vi "ezAFM Practice 1.9.vi"() -> ()   [LabVIEW 2015]
uses:
  LabVIEW for ezAFM/LV-PGC 2019-05a/Universal vi's/Controls/RoboProbe/RoboProbe ID.ctl
  LabVIEW for ezAFM/LV-PGC 2019-05a/Universal vi's/Controls/RoboProbe/RoboProbe PadResults.ctl
  LabVIEW for ezAFM/LV-PGC 2019-05a/Universal vi's/Controls/RoboProbe/RoboProbe DeviceTypes.ctl
  <vilib>/userdefined/High Color/IMAQdx.ctl
  D:/LabVIEW for ezAFM/LV-PGC 2019-05a/Special Equipment/ezAFM/NMI Integration Code/ezCommander.dll
  LabVIEW for ezAFM/LV-PGC 2019-05a/Special Equipment/ezAFM/NMI Integration Code/ezCommander.dll
  LabVIEW for ezAFM/LV-PGC 2019-05a/Universal vi's/Global Variables/Globals-EasyAFM.vi
  Helper VI's/Globals.vi
  <vilib>/vision/driver/NI_Vision_Acquisition_Software.lvlib
panel:
  in  "Update Device List":bool
  out "List of Connections":string[](array[string])
  out "Selected \nConnections":T1[](array[typedef]) {"Results"."Rpad" format="%_2e"; "Results"."S" format="%_2g"; "Results"."Vt" format="%.1f"; "Results"."DV" format="%.2g"; "Results"."Ron" format="%.2e"; "Results"."Roff" format="%.2g"; "Results"."Vg-off" format="%.2g"; "Results"."Vg-on" format="%.2g"; "Results"."DG%" format="%.1f"; "Results"."Gon" format="%.2e"; "Results"."Goff" format="%.2e"; "Results"."Rgate" format="%.2e"; "Results"."I offset" format="%.2e"; "G(Vg)" format="%#_2e"; "ID"."Die" items=["AD", "AE", "AF", "AG", "AH", "AI", "AJ", "BC", "BD", "BE", "BF", "BG", "BH", "BI", "BJ", "BK", "CB", "CC", "CD", "CE", "CF", "CG", "CH", "CI", "CJ", "CK", "CL", "DA", "DB", "DC", "DD", "DE", "DF", "DG", "DH", "DI", "DJ", "DK", "DL", "DM", "EA", "EB", "EC", "ED", "EE", "EF", "EG", "EH", "EI", "EJ", "EK", "EL", "EM", "FA", "FB", "FC", "FD", "FE", "FF", "FG", "FH", "FI", "FJ", "FK", "FL", "FM", "GA", "GB", "GC", "GD", "GE", "GF", "GG", "GH", "GI", "GJ", "GK", "GL", "GM", "HA", "HB", "HC", "HD", "HE", "HF", "HG", "HH", "HI", "HJ", "HK", "HL", "HM", "IA", "IB", "IC", "ID", "IE", "IF", "IG", "IH", "II", "IJ", "IK", "IL", "IM", "JB", "JC", "JD", "JE", "JF", "JG", "JH", "JI", "JJ", "JK", "JL", "KC", "KD", "KE", "KF", "KG", "KH", "KI", "KJ", "KK", "LD", "LE", "LF", "LG", "LH", "LI", "LJ"]; "ID"."Leads" items=["ab", "bc", "cd", "de", "ef", "fg", "gh", "ac", "ce", "eg", "bd", "df", "fh"]; "ID"."Device#" items=["00", "01", "02", "03", "10", "11", "12", "13", "20", "21", "22", "23", "30", "31", "32", "33"]; "Date" format="%<%H:%M\n%d/%m/%y>T"}
  out "Scan Spot Coordinates":dbl[](array[numeric])
  out "Name":string
  out "Sequence Index":dbl
  out "Direction":dbl
  out "Crosshair Found?":bool
  in  "Search":bool
  out "Total Steps":dbl
  out "Current Steps":dbl
  in  "Camera":enum32{"ezAFM Camera"}(tab)
  out "ezAFM Camera":T4(plugin-control)
  in  "Connection to Scan":string
  in  "Initialize Automatic \nRepositioning":bool
  out "Imaging Status":string
  out "Automated Imaging":bool
  in  "Main Menu":T5(tab)
  in  "Navigation Buttons":T6
  in  "Motor Speed":u16(ring)=30000 items=["SLOW"=3300, "MEDIUM"=30000, "FAST"=65000]
  in  "Target Crosshair":string(combo)="00 | 01"
  in  "Current Crosshair":string(combo)="00 | 01"
  in  "MOVE2CROSSHAIR":bool
  in  "THETA":bool
  in  "Angle":dbl
  in  "Step Size":dbl
  in  "Scan Spot":string(combo)
  in  "MOVE2SCANSPOT":bool
  in  "RETRACT":bool
  in  "APPROACH":bool
  in  "SEARCH":bool
  in  "SCAN":bool
  in  "REMOVE":bool
  out "Sequence":string[](array[string])
  in  "Initialize Automated Imaging":bool
  in  "SELECT":bool
  in  "DeviceList":i32(listbox) caption="Devices Selected for AFM Imaging"
  in  "ezAFM Default File Path":path=path "D:/ezAFM/Scanned Images"
  in  "Saved Images File Path":path=path "D:/ezAFM/Scanned Images"
  in  "Wafer Type":string(combo)
  in  "Die":string(combo)
  in  "Image Resolution":u16(ring)=256 items=["128"=128, "256"=256, "512"=512, "1024"=1024]
  in  "Indicators":enum32{"Indicators"}(tab)
  out "XYZ Motor Position":dbl[](array[numeric]) format="%#_4f"
  out "ezAFM Status":dbl
  out "Approaching":bool
  out "ezAFM Connected":bool
  out "Retracting":bool
  out "Scanning":bool
  out "Tip Approached?":bool
  in  "RESET":bool
  out "XY Position":dbl[](array[numeric])
  in  "QUIT":bool
  out "Searching":bool
  # "ON"
  # "OFF"
  # "Use Arrow Keys to manually\nmove the XY Motor"
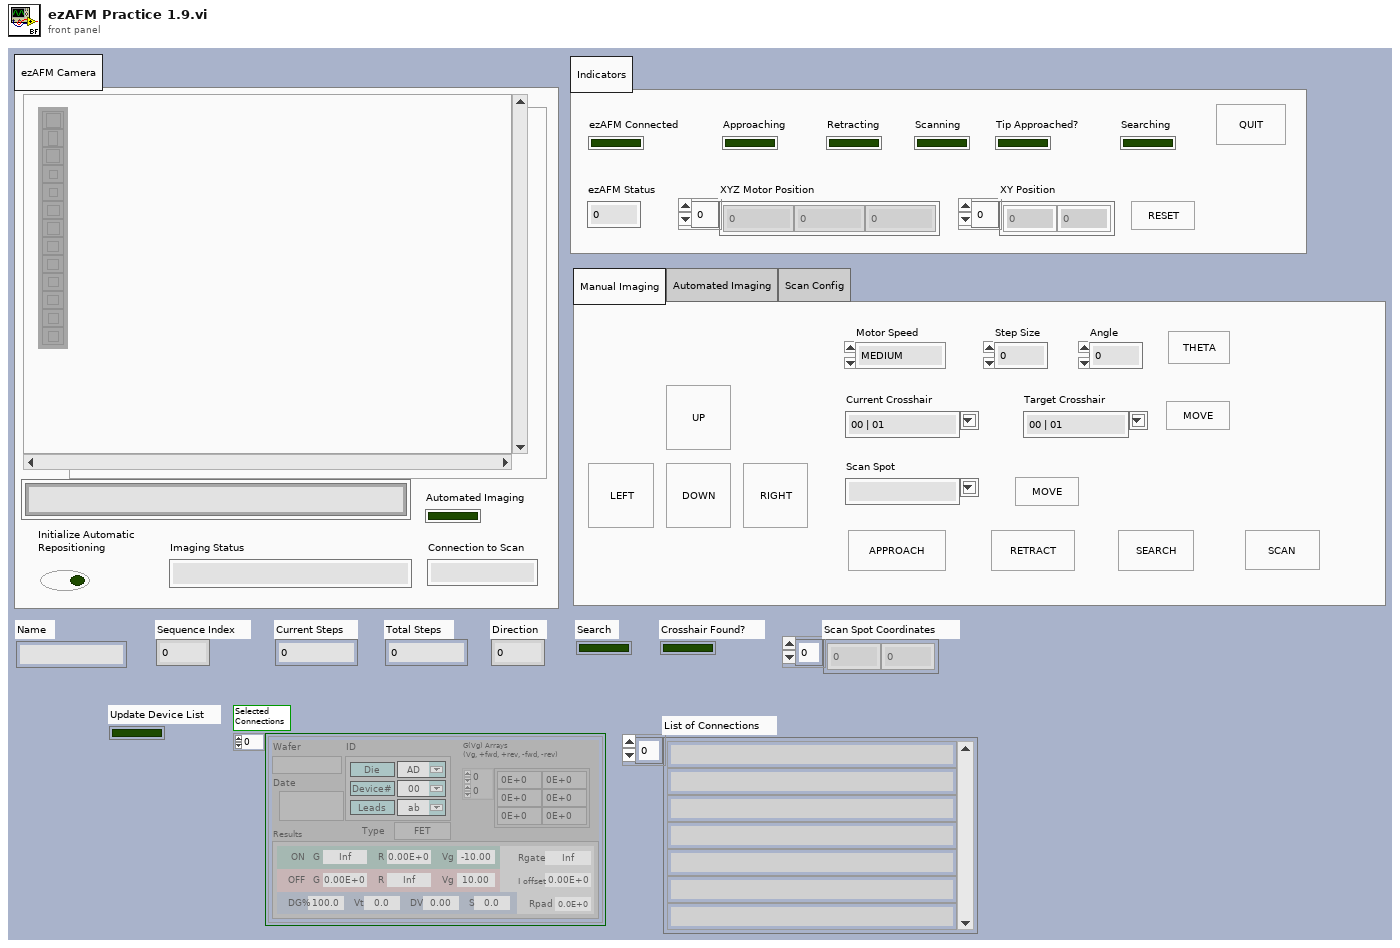
[diagram p1: front panel]
types:
  T1 = typedef "RoboProbe ID.ctl" = cluster{"Wafer":string, "Date":timestamp, "ID":cluster{"Device#":u16, "Leads":u16, "Die":u16}, "G(Vg)":sgl[][], "Results":T2, "Type":T3}
  T2 = typedef "RoboProbe PadResults.ctl" = cluster{"I offset":sgl, "Rgate":sgl, "Gon":sgl, "Goff":sgl, "DG%":sgl, "Ron":sgl, "Vg-on":sgl, "Roff":sgl, "Vg-off":sgl, "DV":sgl, "Vt":sgl, "S":sgl, "Rpad":sgl}
  T3 = typedef "RoboProbe DeviceTypes.ctl" = enum16{"FET", "Metal", "Mixed", "GateLeak", "ShortCirc", "Open", "Untested"}
  T4 = typedef "IMAQ Image.ctl" = refnum<image>
  T5 = enum32{"Manual Imaging", "Automated Imaging", "Scan Config"}
  T6 = cluster{"UP":bool, "DOWN":bool, "LEFT":bool, "RIGHT":bool}
  T7 = typedef "IMAQdx.ctl" = refnum<k21>
  T8 = typedef "Image Type" = u32
  T9 = typedef "eventvkey.ctl" = enum16{"ASCII", "Enter", "Return", "Shift", "Ctrl", "Alt", "Cmd", "Opt", "Caps", "NumLock", "Clear", "Break", "Up", "Down", "Left", "Right", "Insert", "Delete", "Home", "End", "PageUp", "PageDown", "Escape", "Help", "Pause", "ScrollLock", "F1", "F2", "F3", "F4", "F5", "F6", "F7", "F8", "F9", "F10", "F11", "F12", "F13", "F14", "F15", "F16", "F17", "F18", "F19", "F20", "F21", "F22", "F23", "F24", "Play", "VolumeUp", "VolumeDown", "Mute", "Two Byte Char"}
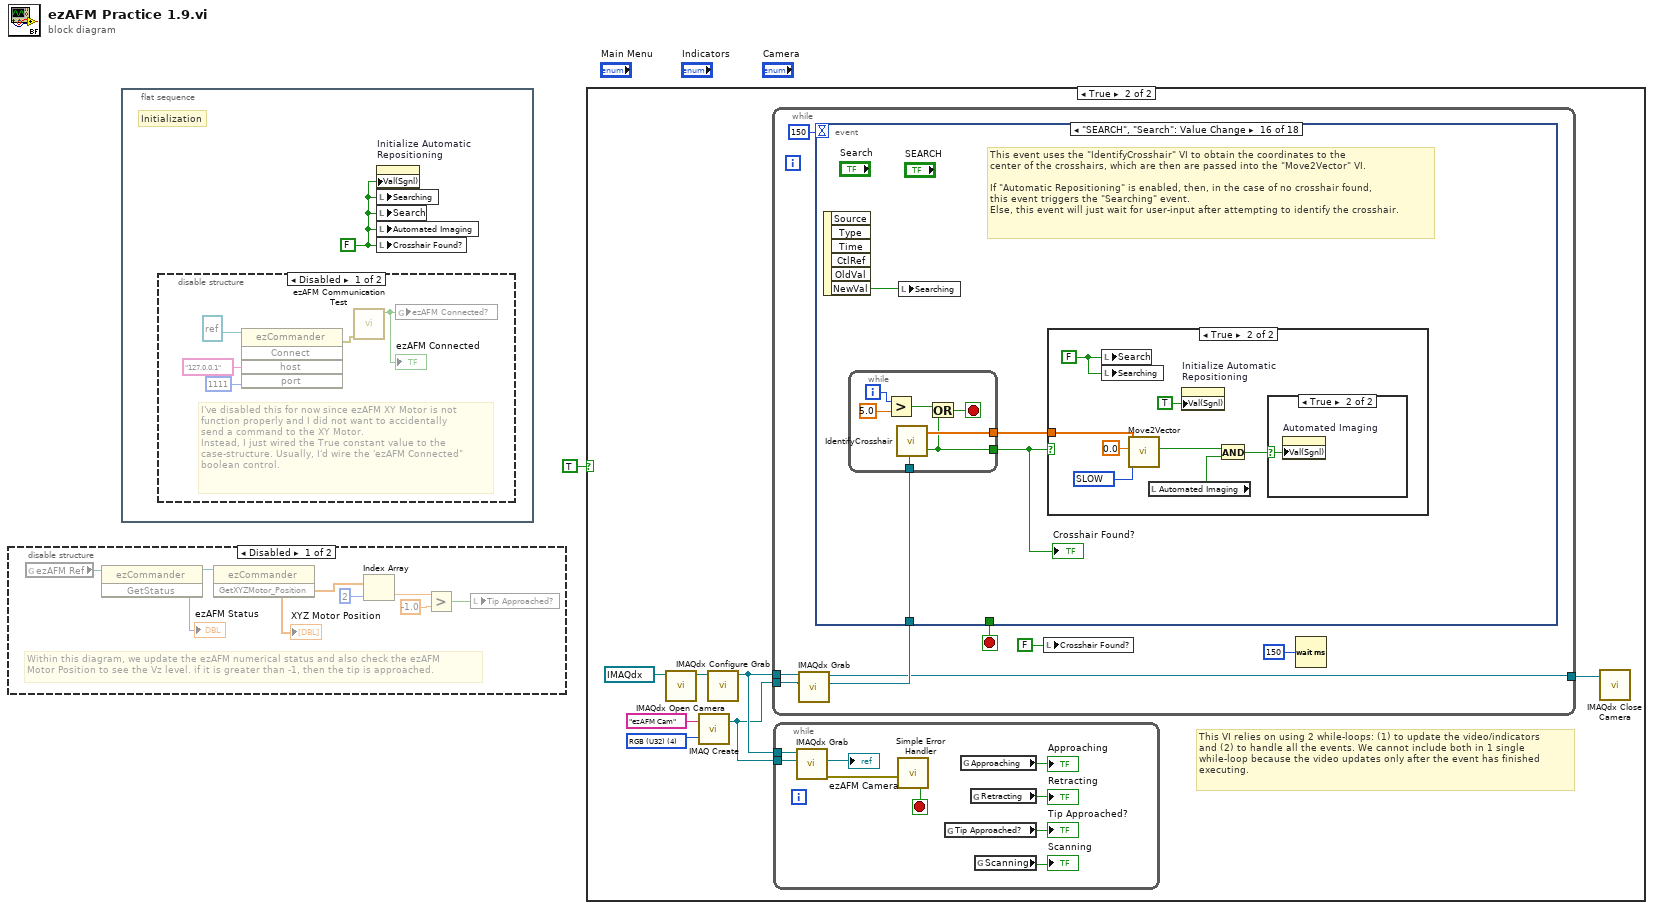
[diagram p0: block diagram]
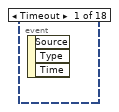
[diagram p5: hidden frame]
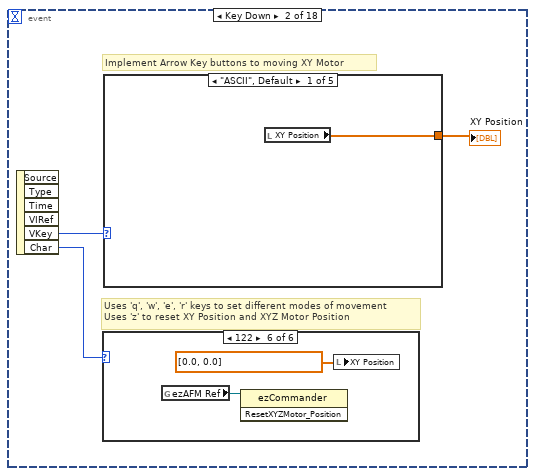
[diagram p6: hidden frame]
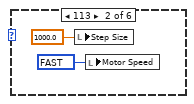
[diagram p8: hidden frame]
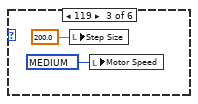
[diagram p9: hidden frame]
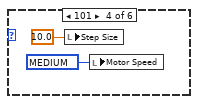
[diagram p10: hidden frame]
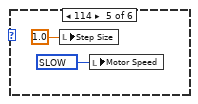
[diagram p11: hidden frame]
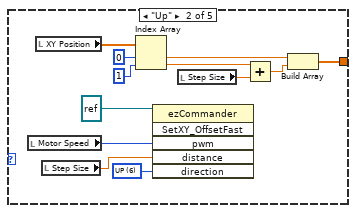
[diagram p12: hidden frame]
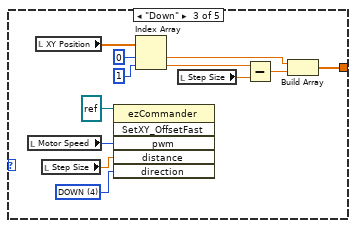
[diagram p13: hidden frame]
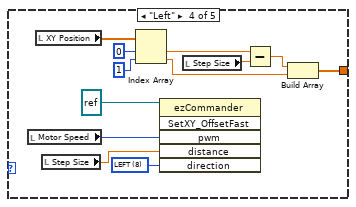
[diagram p14: hidden frame]
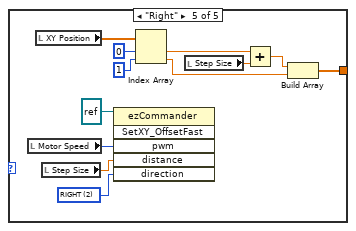
[diagram p15: hidden frame]
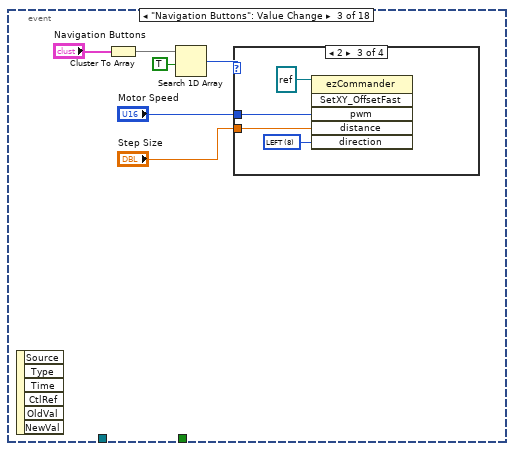
[diagram p16: hidden frame]
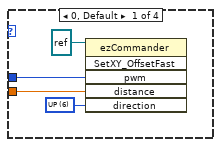
[diagram p17: hidden frame]
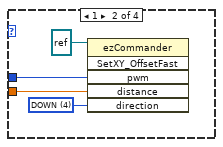
[diagram p18: hidden frame]
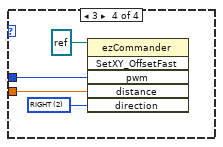
[diagram p19: hidden frame]
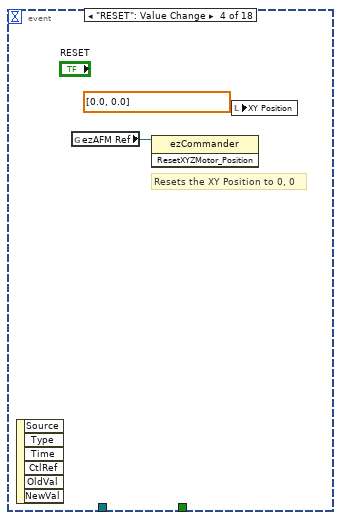
[diagram p20: hidden frame]
diagram:
  n1 = disable-structure shown="Disabled" {
    frame Disabled {
      # "Within this diagram, we update the ezAFM numerical status and also check the ezAFM\nMotor Position to see the Vz level. if it is greater than -1, then the tip is approached."
      n2 = global read "Globals-EasyAFM.vi" "ezAFM Ref"() -> (w7:refnum<k24>)
      n3 = invoke class="ezCommander" method="GetStatus"(reference=w7) -> (reference out=w5:refnum<k24>, "GetStatus"=→"ezAFM Status":i32)  [unwired: 2 in, 1 out]
      n4 = invoke class="ezCommander" method="GetXYZMotor_Position"(reference=w5) -> ("GetXYZMotor_Position"=w9:dbl[])  [unwired: 2 in, 2 out]
      "XYZ Motor Position" <- w9
      n5 = Index Array(array=w9, index=2) -> (element=w4:dbl)
      n6 = Greater?(x=w4, y=-1.0) -> (0:w8:bool)
      n7 = local write "Tip Approached?"(w8) -> ()
    }
    frame Enabled {
    }
  }
  n8 = flat-sequence {
    frame #0 {
      w10 = FALSE ("Automated Imaging")
      # "Initialization"
      n9 = disable-structure shown="Disabled" {
        frame Disabled {
          # "I've disabled this for now since ezAFM XY Motor is not \nfunction properly and I did not want to accidentally\nsend a command to the XY Motor. \nInstead, I just wired the True constant value to the \ncase-structure. Usually, I'd wire the 'ezAFM Connected\"\nboolean control."
          n10 = invoke class="ezCommander" method="Connect"(reference=refnum<k24> refnum ("ezAFM Ref"), "host"="127.0.0.1", "port"=1111) -> (error out=w14:errorcluster)  [unwired: 2 in, 4 out]
          n11 = call "ezAFM Communication Test.vi"("error in"=w14) -> ("ezAFM COM status"=w11:bool)  [unwired: 3 in, 3 out]
          "ezAFM Connected" <- w11
          n12 = global write "Globals.vi" "ezAFM Connected?"(w11) -> ()
        }
        frame Enabled {
        }
      }
      n13 = property on="Initialize Automatic \nRepositioning" class="Bool (strict)"("Val(Sgnl)"=w10) -> ()  [unwired: 2 in, 2 out]
      n14 = local write "Searching"(w10) -> ()
      n15 = local write "Search"(w10) -> ()
      n16 = local write "Automated Imaging"(w10) -> ()
      n17 = local write "Crosshair Found?"(w10) -> ()
    }
  }
  n18 = case shown="True" TRUE {
    frame False {
    }
    frame True {
      w19 = T8 4 items=["Grayscale (U8)", "Grayscale (I16)", "Grayscale (SGL)", "Complex (CSG)", "RGB (U32)", "HSL (U32)", "RGB (U64)", "Grayscale (U16)"] ("Image Type")
      # "This VI relies on using 2 while-loops: (1) to update the video/indicators \nand (2) to handle all the events. We cannot include both in 1 single \nwhile-loop because the video updates only after the event has finished \nexecuting."
      n19 = call <vilib>:"IMAQdx Open Camera.vi"("Session In"=T7 "cam5") -> ("Session Out"=w20:T7)  [unwired: 9 in, 1 out]
      n20 = call "IMAQ Create"("Image Name"="ezAFM Cam", "Image Type"=w19) -> ("New Image"=w17:T4)  [unwired: 3 in, 1 out]
      n21 = call <vilib>:"IMAQdx Configure Grab.vi"("Session In"=w20) -> ("Session Out"=w18:T7)  [unwired: 9 in, 1 out]
      n22 = while {
        tunnel: w18 -> [w37]
        tunnel: w17 -> [w36]
        tunnel: [w34] -> w16
        stop <- w33 stop-if-true
        n23 = call <vilib>:"IMAQdx Grab.vi"("Image In"=w36, "Session In"=w37) -> ("Image Out"=w35:T4, "Session Out"=w34:T7)  [unwired: 2 in, 6 out]
        n24 = event shown="[15] \"SEARCH\", \"Search\": Value Change" {
          selector: _ -> [_ _ _ _ _ _ _ _ _ _ _ _ _ _ _ _ _ _]
          dyn-events: _ -> [_ _ _ _ _ _ _ _ _ _ _ _ _ _ _ _ _ _]
          timeout: 150 -> [_ _ _ _ _ _ _ _ _ _ _ _ _ _ _ _ _ _]
          tunnel: [_ _ _ _ _ _ _ _ _ _ _ _ _ _ _ _ _ "QUIT"] -> w33
          tunnel: w35 -> [_ _ _ _ _ _ _ _ _ _ _ _ _ _ _ w307 _ _]
          event Timeout {
            n25 = event-data() -> ()  [unwired: 1 in, 3 out]
          }
          event Key Down {
            # "Uses 'q', 'w', 'e', 'r' keys to set different modes of movement\nUses 'z' to reset XY Position and XYZ Motor Position"
            # "Implement Arrow Key buttons to moving XY Motor"
            n26 = event-data() -> ("VKey"=w40:T9, "Char"=w41:i16)  [unwired: 1 in, 4 out]
            n27 = case shown="122" w41 {
              frame 0, Default {
              }
              frame 113 {
                w43 = u16 65000 items=["SLOW"=3300, "MEDIUM"=30000, "FAST"=65000] ("Motor Speed")
                n28 = local write "Step Size"(1000.0 ("Step Size")) -> ()
                n29 = local write "Motor Speed"(w43) -> ()
              }
              frame 119 {
                w45 = u16 30000 items=["SLOW"=3300, "MEDIUM"=30000, "FAST"=65000] ("Motor Speed")
                n30 = local write "Step Size"(200.0 ("Step Size")) -> ()
                n31 = local write "Motor Speed"(w45) -> ()
              }
              frame 101 {
                w47 = u16 30000 items=["SLOW"=3300, "MEDIUM"=30000, "FAST"=65000] ("Motor Speed")
                n32 = local write "Step Size"(10.0 ("Step Size")) -> ()
                n33 = local write "Motor Speed"(w47) -> ()
              }
              frame 114 {
                w49 = u16 3300 items=["SLOW"=3300, "MEDIUM"=30000, "FAST"=65000] ("Motor Speed")
                n34 = local write "Step Size"(1.0 ("Step Size")) -> ()
                n35 = local write "Motor Speed"(w49) -> ()
              }
              frame 122 {
                n36 = global read "Globals-EasyAFM.vi" "ezAFM Ref"() -> (w51:refnum<k24>)
                n37 = invoke class="ezCommander" method="ResetXYZMotor_Position"(reference=w51) -> ()  [unwired: 2 in, 3 out]
                n38 = local write "XY Position"(dbl[] [0.0, 0.0] ("XY Position")) -> ()
              }
            }
            n39 = case shown="\"ASCII\", Default" w40 {
              tunnel: [w53 w55 w66 w78 w90] -> w42
              frame "ASCII", Default {
                n40 = local read "XY Position"() -> (w53:dbl[])
              }
              frame "Up" {
                w64 = u16 6 items=["UP"=6, "DOWN"=4, "LEFT"=8, "RIGHT"=2]
                n41 = local read "Motor Speed"() -> (w63:u16)
                n42 = local read "XY Position"() -> (w61:dbl[])
                n43 = local read "Step Size"() -> (w62:dbl)
                n44 = Index Array(array=w61, index #1=0 ("index"), index #2=1 ("index")) -> (element #1=w57:dbl, element #2=w54:dbl)
                n45 = invoke class="ezCommander" method="SetXY_OffsetFast"(reference=refnum<k24> refnum ("ezAFM Ref"), "pwm"=w63, "distance"=w62, "direction"=w64) -> ()  [unwired: 2 in, 6 out]
                n46 = local read "Step Size"() -> (w58:dbl)
                n47 = Add(x=w54, y=w58) -> (x+y=w56:dbl)
                n48 = Build Array(w57, w56) -> (w55:dbl[])
              }
              frame "Down" {
                w74 = u16 4 items=["UP"=6, "DOWN"=4, "LEFT"=8, "RIGHT"=2]
                n49 = local read "Motor Speed"() -> (w76:u16)
                n50 = local read "XY Position"() -> (w68:dbl[])
                n51 = local read "Step Size"() -> (w75:dbl)
                n52 = invoke class="ezCommander" method="SetXY_OffsetFast"(reference=refnum<k24> refnum ("ezAFM Ref"), "pwm"=w76, "distance"=w75, "direction"=w74) -> ()  [unwired: 2 in, 6 out]
                n53 = Index Array(array=w68, index #1=0 ("index"), index #2=1 ("index")) -> (element #1=w70:dbl, element #2=w71:dbl)
                n54 = local read "Step Size"() -> (w67:dbl)
                n55 = Subtract(x=w71, y=w67) -> (x-y=w69:dbl)
                n56 = Build Array(w70, w69) -> (w66:dbl[])
              }
              frame "Left" {
                w88 = u16 8 items=["UP"=6, "DOWN"=4, "LEFT"=8, "RIGHT"=2]
                n57 = local read "Motor Speed"() -> (w86:u16)
                n58 = local read "XY Position"() -> (w82:dbl[])
                n59 = local read "Step Size"() -> (w87:dbl)
                n60 = Index Array(array=w82, index #1=0 ("index"), index #2=1 ("index")) -> (element #1=w81:dbl, element #2=w79:dbl)
                n61 = invoke class="ezCommander" method="SetXY_OffsetFast"(reference=refnum<k24> refnum ("ezAFM Ref"), "pwm"=w86, "distance"=w87, "direction"=w88) -> ()  [unwired: 2 in, 6 out]
                n62 = local read "Step Size"() -> (w83:dbl)
                n63 = Subtract(x=w81, y=w83) -> (x-y=w80:dbl)
                n64 = Build Array(w80, w79) -> (w78:dbl[])
              }
              frame "Right" {
                w100 = u16 2 items=["UP"=6, "DOWN"=4, "LEFT"=8, "RIGHT"=2]
                n65 = local read "Motor Speed"() -> (w99:u16)
                n66 = local read "XY Position"() -> (w95:dbl[])
                n67 = local read "Step Size"() -> (w98:dbl)
                n68 = invoke class="ezCommander" method="SetXY_OffsetFast"(reference=refnum<k24> refnum ("ezAFM Ref"), "pwm"=w99, "distance"=w98, "direction"=w100) -> ()  [unwired: 2 in, 6 out]
                n69 = Index Array(array=w95, index #1=0 ("index"), index #2=1 ("index")) -> (element #1=w93:dbl, element #2=w91:dbl)
                n70 = local read "Step Size"() -> (w94:dbl)
                n71 = Add(x=w93, y=w94) -> (x+y=w92:dbl)
                n72 = Build Array(w92, w91) -> (w90:dbl[])
              }
            }
            "XY Position" <- w42
          }
          event "Navigation Buttons": Value Change {
            n73 = event-data() -> ()  [unwired: 1 in, 6 out]
            n74 = Cluster To Array(cluster="Navigation Buttons") -> (array=w106:bool[])
            n75 = Search 1D Array(1D array=w106, element=TRUE) -> (index of element=w104:i32)  [unwired: 1 in]
            n76 = case shown="2" w104 {
              tunnel: "Step Size" -> [w108 w113 w117 w121]
              tunnel: "Motor Speed" -> [w109 w112 w116 w120]
              frame 0, Default {
                w110 = u16 6 items=["UP"=6, "DOWN"=4, "LEFT"=8, "RIGHT"=2]
                n77 = invoke class="ezCommander" method="SetXY_OffsetFast"(reference=refnum<k24> refnum ("ezAFM Ref"), "pwm"=w109, "distance"=w108, "direction"=w110) -> ()  [unwired: 2 in, 6 out]
              }
              frame 1 {
                w114 = u16 4 items=["UP"=6, "DOWN"=4, "LEFT"=8, "RIGHT"=2]
                n78 = invoke class="ezCommander" method="SetXY_OffsetFast"(reference=refnum<k24> refnum ("ezAFM Ref"), "pwm"=w112, "distance"=w113, "direction"=w114) -> ()  [unwired: 2 in, 6 out]
              }
              frame 2 {
                w118 = u16 8 items=["UP"=6, "DOWN"=4, "LEFT"=8, "RIGHT"=2]
                n79 = invoke class="ezCommander" method="SetXY_OffsetFast"(reference=refnum<k24> refnum ("ezAFM Ref"), "pwm"=w116, "distance"=w117, "direction"=w118) -> ()  [unwired: 2 in, 6 out]
              }
              frame 3 {
                w122 = u16 2 items=["UP"=6, "DOWN"=4, "LEFT"=8, "RIGHT"=2]
                n80 = invoke class="ezCommander" method="SetXY_OffsetFast"(reference=refnum<k24> refnum ("ezAFM Ref"), "pwm"=w120, "distance"=w121, "direction"=w122) -> ()  [unwired: 2 in, 6 out]
              }
            }
          }
          event "RESET": Value Change {
            # "Resets the XY Position to 0, 0"
            n81 = event-data() -> ()  [unwired: 1 in, 6 out]
            n82 = global read "Globals-EasyAFM.vi" "ezAFM Ref"() -> (w124:refnum<k24>)
            n83 = invoke class="ezCommander" method="ResetXYZMotor_Position"(reference=w124) -> ()  [unwired: 2 in, 3 out]
            n84 = local write "XY Position"(dbl[] [0.0, 0.0] ("XY Position")) -> ()
          }
          event "THETA": Value Change {
            # "NOTE: 9/17/2019: This feature does not work reliably because XY Position is a simple record of horizontal\nand vertical movements without accounting for Motor Speed. Different Motor Speeds lead to different\nerror and physical distance values.\nI've noticed that using any generic angle measurement tool such as Windows Snip and entering the estimated angle\ninto the control value works sufficiently."
            # "Takes the absolute value of the XY Position and computes the magnitude of the angle.\nThen based on the sign of the X and Y position, we change the sign of the angle\nIf both signs are the same, then the angle should be negative (clockwise rotated by theta)\nElse if both signs are different, then the angle should be positive (counter-clockwise rotated)"
            n85 = event-data() -> ()  [unwired: 1 in, 6 out]
            n86 = local read "XY Position"() -> (w139:dbl[])
            n87 = Absolute Value(x=w139) -> (abs(x)=w140:dbl[])
            n88 = Index Array(array=w139) -> (element #1=w133:dbl, element #2=w132:dbl)  [unwired: 2 in]
            n89 = Index Array(array=w140, index #1=1 ("index"), index #2=0 ("index")) -> (element #1=w136:dbl, element #2=w135:dbl)
            n90 = Re/Im To Complex(1:w135, 2:w136) -> (0:w134:cdb)
            n91 = Sign(1:w133) -> (0:w131:dbl)
            n92 = Sign(1:w132) -> (0:w130:dbl)
            n93 = Complex To Polar(r * e^(i*theta)=w134) -> (theta=w128:dbl)  [unwired: 1 out]
            n94 = Equal?(x=w131, y=w130) -> (x = y?=w129:bool)
            n95 = case shown="True" w129 {
              tunnel: w128 -> [w141 w143]
              tunnel: [w141 w142] -> w127
              frame False {
              }
              frame True {
                n96 = Negate(x=w143) -> (-x=w142:dbl)
              }
            }
            n97 = expression code="(x/pi)*180.0" "radians to degrees"(w127) -> (w126:dbl)
            n98 = local write "Angle"(w126) -> ()
            n99 = global write "Globals.vi" "THETA"(w126) -> ()
          }
          event "APPROACH", "RETRACT": Value Change {
            n100 = event-data() -> ()  [unwired: 1 in, 6 out]
            n101 = case shown="True" "APPROACH" {
              selector: "APPROACH" -> [_ w149]
              frame False {
              }
              frame True {
                n102 = call "AutoLand&Approach.vi"("Autoland?"=w149, "Step-Approach?"=FALSE) -> ()  [unwired: 1 out]
              }
            }
            n103 = case shown="True" "RETRACT" {
              selector: "RETRACT" -> [_ w146]
              frame False {
              }
              frame True {
                n104 = call "Retract.vi"("Number of Cycles"=10, "Retracting?"=w146) -> ()  [unwired: 1 out]
              }
            }
          }
          event "SELECT", "REMOVE": Value Change {
            # "This event handles selecting/removing connections to scan.\nI copied/pasted this from Trevor's \"ezAFM Automated Imaging 3.3\"\n\n10/6/2019: There are some file errors (\"Device Config\") with the \"SimpleMap\" VI"
            n105 = event-data() -> ()  [unwired: 1 in, 6 out]
            n106 = case shown="True" "SELECT" {
              frame False {
              }
              frame True {
                n107 = call "SimpleMap.vi"() -> ("Selected Connections"=→"Selected \nConnections":T1[])  [unwired: 5 in, 2 out]
              }
            }
            n108 = case shown="True" "REMOVE" {
              tunnel: "DeviceList" -> [_ w154]
              frame False {
              }
              frame True {
                n109 = local read "Selected \nConnections"() -> (w155:T1[])
                n110 = Two Button Dialog(message="Press Confirm to remove the selected connections from the queue", 2:"Confirm" ("T button name (\"OK\")")) -> (T button?=w156:bool)  [unwired: 1 in]
                n111 = case shown="True" w156 {
                  tunnel: w154 -> [_ w161]
                  tunnel: w155 -> [_ w160]
                  frame False {
                    # "Do nothing if cancelled"
                  }
                  frame True {
                    n112 = Delete From Array(array=w160, index=w161) -> (array with subset deleted=w159:T1[])  [unwired: 1 in, 1 out]
                    n113 = local write "Selected \nConnections"(w159) -> ()
                  }
                }
              }
            }
            n114 = property on="Update Device List" class="Bool (strict)"("Val(Sgnl)"=TRUE ("Value (Signaling)")) -> ()  [unwired: 2 in, 2 out]
          }
          event "Update Device List": Value Change {
            w169 = 18 ("y")
            # "This for-loop takes in the list of clusters of connections\nand turns it into a simple string array of connections\nwhich is then used for the \"BuildSequence\" VI."
            n115 = event-data() -> ()  [unwired: 1 in, 6 out]
            n116 = local read "Selected \nConnections"() -> (w167:T1[])
            n117 = local read "Selected \nConnections"() -> (w172:T1[])
            n118 = for {
              tunnel: w167 -> [w185] mode=indexing
              shift-right: [w184] -> w168
              shift-left: string[] [] -> [w176]
              n119 = Unbundle By Name(w185) -> ("ID"=w186:cluster{"Device#":u16, "Leads":u16, "Die":u16})
              n120 = property on="Die" class="Ring (strict)"() -> ("Strings []"=w175:string[])  [unwired: 2 in, 2 out]
              n121 = property on="Device#" class="Ring (strict)"() -> ("Strings []"=w174:string[])  [unwired: 2 in, 2 out]
              n122 = property on="Leads" class="Ring (strict)"() -> ("Strings []"=w173:string[])  [unwired: 2 in, 2 out]
              n123 = Unbundle By Name(w186) -> ("Die"=w181:u16, "Device#"=w183:u16, "Leads"=w182:u16)
              n124 = Index Array(array=w175, index=w181) -> (element=w180:string)
              n125 = Index Array(array=w174, index=w183) -> (element=w179:string)
              n126 = Index Array(array=w173, index=w182) -> (element=w178:string)
              n127 = Concatenate Strings(w180, w179, w178) -> (w177:string)
              n128 = Build Array (concatenate)(w176, w177) -> (w184:string[])
            }
            "List of Connections" <- w168
            n129 = call "ezAFM Build ScanList from Connections.vi"("Selected Connections"=w172) -> ("Item Names"=w166:string[][])  [unwired: 1 in, 1 out]
            n130 = Array Size(array=w172) -> (size(s)=w171:i32)
            n131 = Increment(x=w171) -> (x+1=w170:i32)
            n132 = Greater?(x=w170, y=w169) -> (0:w164:bool)
            n133 = Max & Min(x=w169, y=w170) -> (min(x,y)=w165:i32)  [unwired: 1 out]
            n134 = property on="DeviceList" class="MCListbox (strict)"("ItemNames"=w166, "NumRows"=w165, "VScrollVis"=w164) -> ()  [unwired: 2 in, 2 out]
          }
          event "Initialize Automated Imaging": Value Change {
            # "This event initializes the parameters for \"Automated Imaging\".\nIt uses the \"BuildSeqeuence' VI to create a string array of movements.\nAlso, this event enables \"Automatic Repositioning\" to find the crosshair."
            n135 = event-data() -> ()  [unwired: 1 in, 6 out]
            n136 = local read "List of Connections"() -> (w191:string[])
            n137 = call "BuildSequence.vi"("Connections"=w191) -> ("Sequence"=w189:string[])
            "Sequence" <- w189
            n138 = Array Size(array=w189) -> (size(s)=w188:i32)
            n139 = Greater Than 0?(x=w188) -> (x > 0?=w187:bool)
            n140 = local write "Initialize Automatic \nRepositioning"(w187) -> ()
            n141 = local write "Automated Imaging"(w187) -> ()
            n142 = property on="Automated Imaging" class="Bool (strict)"("Val(Sgnl)"=w187) -> ()  [unwired: 2 in, 2 out]
            "Sequence Index" <- -1.0 ("Index")
          }
          event "Automated Imaging": Value Change {
            # "This event is sort of the \"main\" event running the Automated Imaging. It relies on other events such as\n\"MOVE2SCANSPOT\" and \"MOVE2CROSSHAIR\".\nWe test substrings within each step in the Sequence to judge whether to execute Coarse or Fine\nmovement commads."
            # "Iterate through the Sequence array"
            n143 = event-data() -> ()  [unwired: 1 in, 6 out]
            n144 = local read "Sequence Index"() -> (w195:dbl)
            n145 = local read "Sequence"() -> (w193:string[])
            n146 = Increment(x=w195) -> (x+1=w194:dbl)
            n147 = local write "Sequence Index"(w194) -> ()
            n148 = Index Array(array=w193, index=w194) -> (element=w192:string)
            "Imaging Status" <- w192
            n149 = Search/Split String(string=w192, search string/char (-)="Scan Spot") -> (offset of match=w198:i32)  [unwired: 1 in, 2 out]
            n150 = Search/Split String(string=w192, search string/char (-)="Crosshairs") -> (offset of match=w199:i32)  [unwired: 1 in, 2 out]
            n151 = Greater Or Equal To 0?(x=w198) -> (x >= 0?=w197:bool)
            n152 = Greater Or Equal To 0?(x=w199) -> (x >= 0?=w196:bool)
            n153 = case shown="True" w196 {
              tunnel: w192 -> [_ w209]
              frame False {
              }
              frame True {
                n154 = String Subset(string=w209, offset (0)=21, length (rest)=7 ("length (rest)")) -> (substring=w203:string)
                n155 = String Subset(string=w209, offset (0)=10, length (rest)=7 ("length (rest)")) -> (substring=w204:string)
                n156 = String Length(string=w204) -> (length=w205:i32)
                n157 = String Length(string=w203) -> (length=w206:i32)
                n158 = local write "Current Crosshair"(w204) -> ()
                n159 = local write "Target Crosshair"(w203) -> ()
                n160 = Greater Than 0?(x=w205) -> (x > 0?=w207:bool)
                n161 = Greater Than 0?(x=w206) -> (x > 0?=w208:bool)
                n162 = And(x=w207, y=w208) -> (x .and. y?=w202:bool)
                n163 = property on="MOVE2CROSSHAIR" class="Bool (strict)"("Val(Sgnl)"=w202) -> ()  [unwired: 2 in, 2 out]
              }
            }
            n164 = case shown="True" w197 {
              tunnel: w192 -> [_ w222]
              tunnel: w192 -> [_ w214]
              frame False {
              }
              frame True {
                n165 = String Subset(string=w222, offset (0)=18, length (rest)=2 ("length (rest)")) -> (substring=w217:string)
                n166 = String Subset(string=w214, offset (0)=25) -> (substring=w216:string)  [unwired: 1 in]
                n167 = local write "Scan Spot"(w217) -> ()
                n168 = local write "Connection to Scan"(w216) -> ()
                n169 = String Length(string=w217) -> (length=w218:i32)
                n170 = String Length(string=w216) -> (length=w219:i32)
                n171 = Greater Than 0?(x=w218) -> (x > 0?=w220:bool)
                n172 = Greater Than 0?(x=w219) -> (x > 0?=w221:bool)
                n173 = And(x=w220, y=w221) -> (x .and. y?=w215:bool)
                n174 = property on="MOVE2SCANSPOT" class="Bool (strict)"("Val(Sgnl)"=w215) -> ()  [unwired: 2 in, 2 out]
              }
            }
          }
          event "MOVE2CROSSHAIR": Value Change {
            w231 = u16 65000 items=["SLOW"=3300, "MEDIUM"=30000, "FAST"=65000] ("Motor Speed")
            # "After moving to the Target Crosshair, this event triggers the \"Search\" event \ndepending on if 'Enable Automatic Repositioning\" is true.\nNOTE: We would set \"Enable Automatic Repositioning\" to be true in the \"Initialize Automated Imaging\" event."
            # "This event addresses Coarse Navigation.\nIt uses the \"GetCrosshairVector\" VI to generate the \nXY Vector representing the relative distance between the \n\"Current\" and \"Target\" Crosshair pertaining to a pair of devices"
            n175 = event-data() -> ()  [unwired: 1 in, 6 out]
            n176 = call "GetCrosshairVector.vi"("Target Crosshair"="Target Crosshair", "Current Crosshair"="Current Crosshair") -> ("XY Vector"=w226:dbl[])  [unwired: 9 in]
            n177 = local read "Angle"() -> (w230:dbl)
            n178 = call "Move2Vector.vi"("Motor Speed"=w231, "Angle"=w230, "XY Vector"=w226) -> ("Finished?"=w229:bool)  [unwired: 8 in]
            n179 = case shown="True" w229 {
              frame False {
              }
              frame True {
                n180 = local read "Initialize Automatic \nRepositioning"() -> (w234:bool)
                n181 = local read "Target Crosshair"() -> (w233:string)
                n182 = local write "MOVE2CROSSHAIR"(FALSE) -> ()
                n183 = local write "Current Crosshair"(w233) -> ()
                n184 = case shown="True" w234 {
                  selector: w234 -> [_ w235]
                  frame False {
                  }
                  frame True {
                    n185 = property on="Search" class="Bool (strict)"("Val(Sgnl)"=w235) -> ()  [unwired: 2 in, 2 out]
                  }
                }
              }
            }
          }
          event "MOVE2SCANSPOT": Value Change {
            w241 = u16 3300 items=["SLOW"=3300, "MEDIUM"=30000, "FAST"=65000] ("Motor Speed")
            # "This event addresses Fine Navigation.\nIt refers to my other helper VI, called \"GetScanSpot\", to obtain the scan spot \ncoordinates for A0, B0, A1, B1. \nIf \"Automated Imaging\" is enabled, then this event, when finished, triggers the \n\"SCAN\" event. \nElse, this will just wait for user-input after moving to the scan spot."
            n186 = event-data() -> ()  [unwired: 1 in, 6 out]
            n187 = for {
              tunnel: string[] ["X edge even", "X edge odd", "Y edge efgh", "Y edge abcde"] -> [w273] mode=indexing
              tunnel: [w272] -> w244 mode=indexing
              n188 = Current VI's Path() -> (path=w280:path)
              n189 = Strip Path(path=w280) -> (stripped path=w279:path)  [unwired: 1 out]
              n190 = Build Path(base path=w279, name or relative path="GetScanSpot.vi") -> (appended path=w277:path)
              n191 = Open VI Reference(vi path=w277) -> (vi reference=w276:refnum<vi>)  [unwired: 5 in, 1 out]
              n192 = invoke class="VI" method="Ctrl Val.Get"(reference=w276, "Control Name"=w273) -> ("Get Control Value Variant"=w275:variant)  [unwired: 2 in, 3 out]
              n193 = Variant To Data(type=0.0, Variant=w275) -> (data=w272:dbl)  [unwired: 1 in, 1 out]
            }
            n194 = case shown="\"B0\"" "Scan Spot" {
              tunnel: w244 -> [_ w252 w254 w260 w266]
              tunnel: [w246 w247 w253 w259 w265] -> w245
              tunnel: [w246 w247 w253 w259 w265] -> w236
              frame Default {
                w246 = dbl[] [0.0, 0.0] ("XY Vector")
              }
              frame "A0" {
                n195 = Index Array(array=w252, index #1=0 ("index"), index #2=3 ("index")) -> (element #1=w249:dbl, element #2=w248:dbl)
                n196 = Build Array(w249, w248) -> (w247:dbl[])
              }
              frame "B0" {
                n197 = Index Array(array=w254, index #1=0 ("index"), index #2=2 ("index")) -> (element #1=w256:dbl, element #2=w255:dbl)
                n198 = Build Array(w256, w255) -> (w253:dbl[])
              }
              frame "A1" {
                n199 = Index Array(array=w260, index #1=1 ("index"), index #2=3 ("index")) -> (element #1=w262:dbl, element #2=w261:dbl)
                n200 = Build Array(w262, w261) -> (w259:dbl[])
              }
              frame "B1" {
                n201 = Index Array(array=w266, index #1=1 ("index"), index #2=2 ("index")) -> (element #1=w268:dbl, element #2=w267:dbl)
                n202 = Build Array(w268, w267) -> (w265:dbl[])
              }
            }
            "Scan Spot Coordinates" <- w236
            n203 = local read "Angle"() -> (w242:dbl)
            n204 = local read "Automated Imaging"() -> (w240:bool)
            n205 = call "Move2Vector.vi"("Motor Speed"=w241, "Angle"=w242, "XY Vector"=w245) -> ("Finished?"=w239:bool)  [unwired: 8 in]
            n206 = And(x=w239, y=w240) -> (x .and. y?=w238:bool)
            n207 = case shown="True" w238 {
              selector: w238 -> [_ w271]
              frame False {
              }
              frame True {
                n208 = property on="SCAN" class="Bool (strict)"("Val(Sgnl)"=w271) -> ()  [unwired: 2 in, 2 out]
              }
            }
          }
          event "Connection to Scan": Value Change {
            # "This event simply updates the \"Name\" indicator for when we save the image files after\ntaking a scan. (\"Name\" is used as a parameter in the \"TakeScan\" VI)"
            n209 = event-data() -> ()  [unwired: 1 in, 6 out]
            n210 = Concatenate Strings("Wafer Type", "-" ("string"), "Die", "Connection to Scan") -> (→"Name":string)
          }
          event "SCAN": Value Change {
            # "This event take a full scan of the connections (3 21x21 micron images).\nIt relies on using the \"TakeScan\" VI.\nIf \"Automated Imaging\" is enabled, then this event, when finished, will trigger\nthe \"Automated Imaging\" event, where the next step in the sequence will be executed.\nElse, this event will just wait for user-input after taking the scan."
            n211 = event-data() -> ()  [unwired: 1 in, 6 out]
            n212 = local read "Angle"() -> (w291:dbl)
            n213 = local read "Automated Imaging"() -> (w287:bool)
            n214 = local read "Name"() -> (w293:string)
            n215 = call "TakeScan.vi"("Target File Path"="Saved Images File Path", "ezAFM Default Path"="ezAFM Default File Path", "Angle"=w291, "Image Resolution"="Image Resolution", "Name"=w293) -> ("Finished?"=w288:bool)  [unwired: 6 in]
            n216 = And(x=w288, y=w287) -> (x .and. y?=w286:bool)
            n217 = case shown="True" w286 {
              frame False {
              }
              frame True {
                w301 = u16 3300 items=["SLOW"=3300, "MEDIUM"=30000, "FAST"=65000] ("Motor Speed")
                # "Re-center cantilever on crosshair\nNOTE: Subtract 30 to move back 2 regions to original Scan Spot"
                n218 = local read "Scan Spot Coordinates"() -> (w294:dbl[])
                n219 = Negate(x=w294) -> (-x=w295:dbl[])
                n220 = Index Array(array=w295) -> (element #1=w297:dbl, element #2=w298:dbl)  [unwired: 2 in]
                n221 = local read "Angle"() -> (w302:dbl)
                n222 = Subtract(x=w297, y=30.0) -> (x-y=w299:dbl)
                n223 = Build Array(w299, w298) -> (w300:dbl[])
                n224 = call "Move2Vector.vi"("Motor Speed"=w301, "Angle"=w302, "XY Vector"=w300) -> ("Finished?"=w303:bool)  [unwired: 8 in]
                n225 = property on="Automated\nImaging" class="Bool (strict)"("Val(Sgnl)"=w303) -> ()  [unwired: 2 in, 2 out]
              }
            }
          }
          event "Initialize Automatic \nRepositioning": Value Change {
            w304 = u16 6 items=["UP"=6, "DOWN"=4, "LEFT"=8, "RIGHT"=2]
            # "This event initializes the parameters involved for my \"Automatic Repositioning\", \nalgorithm which includes 3 events; this one, \"Search\", and \"Searching\""
            n226 = event-data() -> ()  [unwired: 1 in, 6 out]
            "Total Steps" <- 1.0 ("Total Distance")
            "Current Steps" <- 0.0 ("Current Steps")
            "Direction" <- w304
          }
          event "SEARCH", "Search": Value Change {
            # "This event uses the \"IdentifyCrosshair\" VI to obtain the coordinates to the \ncenter of the crosshairs, which are then are passed into the \"Move2Vector\" VI.\n\nIf \"Automatic Repositioning\" is enabled, then, in the case of no crosshair found,\nthis event triggers the \"Searching\" event.\nElse, this event will just wait for user-input after attempting to identify the crosshair."
            n227 = event-data() -> ("NewVal"=w308:bool)  [unwired: 1 in, 5 out]
            n228 = while {
              tunnel: w307 -> [w317]
              tunnel: [w313] -> w309
              tunnel: [w316] -> w310
              i -> [w314]
              stop <- w311 stop-if-true
              n229 = Greater?(x=w314, y=5.0) -> (0:w312:bool)
              n230 = call "IdentifyCrosshair.vi"("ezAFM Camera"=w317) -> ("Delta"=w316:dbl[], "Found?"=w313:bool)
              n231 = Or(x=w312, y=w313) -> (x .or. y?=w311:bool)
            }
            "Crosshair Found?" <- w309
            n232 = local write "Searching"(w308) -> ()
            n233 = case shown="True" w309 {
              tunnel: w310 -> [_ w328]
              frame False {
                n234 = local read "Initialize Automatic \nRepositioning"() -> (w319:bool)
                n235 = local write "Searching"(FALSE ("Searching")) -> ()
                n236 = case shown="True" w319 {
                  frame False {
                  }
                  frame True {
                    n237 = property on="Searching" class="Bool (strict)"("Val(Sgnl)"=TRUE ("Value (Signaling)")) -> ()  [unwired: 2 in, 2 out]
                  }
                }
              }
              frame True {
                w326 = FALSE ("SEARCH")
                w327 = u16 3300 items=["SLOW"=3300, "MEDIUM"=30000, "FAST"=65000] ("Motor Speed")
                n238 = local write "Search"(w326) -> ()
                n239 = local write "Searching"(w326) -> ()
                n240 = call "Move2Vector.vi"("Motor Speed"=w327, "Angle"=0.0, "XY Vector"=w328) -> ("Finished?"=w322:bool)  [unwired: 8 in]
                n241 = local read "Automated Imaging"() -> (w321:bool)
                n242 = property on="Initialize Automatic \nRepositioning" class="Bool (strict)"("Val(Sgnl)"=TRUE ("Value (Signaling)")) -> ()  [unwired: 2 in, 2 out]
                n243 = And(x=w322, y=w321) -> (x .and. y?=w323:bool)
                n244 = case shown="True" w323 {
                  selector: w323 -> [_ w329]
                  frame False {
                  }
                  frame True {
                    n245 = property on="Automated Imaging" class="Bool (strict)"("Val(Sgnl)"=w329) -> ()  [unwired: 2 in, 2 out]
                  }
                }
              }
            }
          }
          event "Searching": Value Change {
            # "At the end of the movement, this event triggers the \n\"Search\" event to atttempt to identify the crosshair."
            # "This event takes in the parameters for \"Automatic Repositioning and sends commands to the\nXY Motor to move in a certain direction. \nThe overall pattern of movement resembles a square spiral."
            n246 = event-data() -> ()  [unwired: 1 in, 6 out]
            n247 = local read "Total Steps"() -> (w332:dbl)
            n248 = local read "Current Steps"() -> (w333:dbl)
            n249 = local read "Direction"() -> (w334:dbl)
            n250 = Equal?(x=w332, y=w333) -> (x = y?=w335:bool)
            n251 = case shown="False" w335 {
              tunnel: w333 -> [w340 _]
              tunnel: w334 -> [w341 w350]
              tunnel: w332 -> [w336 w346]
              tunnel: [TRUE ("Value (Signaling)") TRUE ("Value (Signaling)")] -> w331
              tunnel: [w336 w345] -> w330
              frame False {
                w342 = u16 65000 items=["SLOW"=3300, "MEDIUM"=30000, "FAST"=65000] ("Motor Speed")
                n252 = Increment(x=w340) -> (x+1=w339:dbl)
                n253 = local write "Current Steps"(w339) -> ()
                n254 = invoke class="ezCommander" method="SetXY_OffsetFast"(reference=refnum<k24> refnum ("ezAFM Ref"), "pwm"=w342, "distance"=20.0, "direction"=w341) -> ()  [unwired: 2 in, 6 out]
                n255 = Wait (ms)(milliseconds to wait=u32 1000) -> ()  [unwired: 1 out]
              }
              frame True {
                n256 = case shown="6" w350 {
                  tunnel: [u16 0 w353 w354 w355 w356] -> w349
                  frame Default {
                  }
                  frame 6 {
                    w353 = u16 2 items=["UP"=6, "DOWN"=4, "LEFT"=8, "RIGHT"=2]
                  }
                  frame 4 {
                    w354 = u16 8 items=["UP"=6, "DOWN"=4, "LEFT"=8, "RIGHT"=2]
                  }
                  frame 8 {
                    w355 = u16 6 items=["UP"=6, "DOWN"=4, "LEFT"=8, "RIGHT"=2]
                  }
                  frame 2 {
                    w356 = u16 4 items=["UP"=6, "DOWN"=4, "LEFT"=8, "RIGHT"=2]
                  }
                }
                n257 = local write "Current Steps"(0.0 ("Current Steps")) -> ()
                n258 = local write "Direction"(w349) -> ()
                n259 = Increment(x=w346) -> (x+1=w345:dbl)
                n260 = Wait (ms)(milliseconds to wait=u32 1000) -> ()  [unwired: 1 out]
              }
            }
            n261 = property on="Search" class="Bool (strict)"("Val(Sgnl)"=w331) -> ()  [unwired: 2 in, 2 out]
            n262 = local write "Total Steps"(w330) -> ()
          }
          event "QUIT": Value Change {
            w358 = FALSE ("ezAFM Connected?")
            n263 = event-data() -> ()  [unwired: 1 in, 6 out]
            n264 = global write "Globals.vi" "ezAFM Connected?"(w358) -> ()
            n265 = local write "ezAFM Connected"(w358) -> ()
          }
        }
        n266 = local write "Crosshair Found?"(FALSE ("Scan")) -> ()
        n267 = Wait (ms)(milliseconds to wait=u32 150) -> ()  [unwired: 1 out]
      }
      n268 = while {
        tunnel: w18 -> [w31]
        tunnel: w17 -> [w30]
        stop <- w27 stop-if-true
        n269 = call <vilib>:"IMAQdx Grab.vi"("Image In"=w30, "Session In"=w31) -> ("error out"=w28:errorcluster, "Image Out"=→"ezAFM Camera":T4)  [unwired: 2 in, 6 out]
        n270 = call <vilib>:"Simple Error Handler.vi"("error in (no error)"=w28) -> ("error?"=w27:bool)  [unwired: 4 in, 4 out]
        n271 = global read "Globals.vi" "Tip Approached?"() -> (→"Tip Approached?":bool)
        n272 = global read "Globals.vi" "Approaching"() -> (→"Approaching":bool)
        n273 = global read "Globals.vi" "Retracting"() -> (→"Retracting":bool)
        n274 = global read "Globals.vi" "Scanning"() -> (→"Scanning":bool)
      }
      n275 = call <vilib>:"IMAQdx Close Camera.vi"("Session In"=w16) -> ()  [unwired: 10 in, 1 out]
    }
  }
